vi "save.vi"(8 "error in (no error)":errorcluster caption="entrée d'erreur (pas d'erreur)", 11 "Model.lvclass":refnum<class "Model.lvclass">) -> (0 "error out":errorcluster caption="sortie d'erreur", 2 "filename":string, 3 "Model.lvclass 2":refnum<class "Model.lvclass">)   [LabVIEW 2020, in "Model.lvclass"]
doc: "Save a trained model"
uses:
  Model.lvclass
  C:/Users/cipop/TDF Dropbox/2_Technologies de France/1 - Services et Etudes/PLAIY/2 - DEV/PLAIYLAB/code/Python/Python.lvclass
  Model.lvclass/Model.ctl
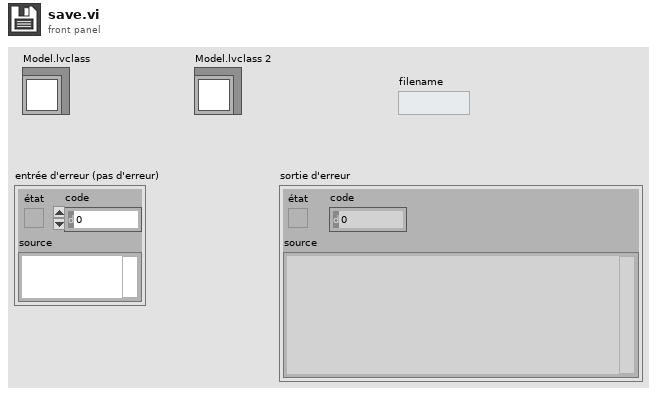
[diagram p1: front panel]
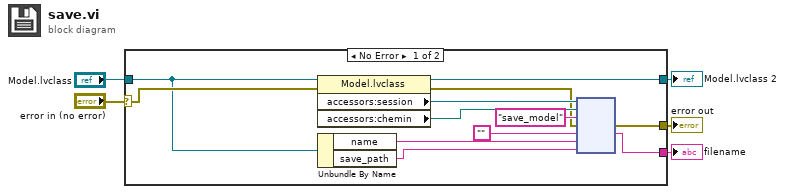
[diagram p0: block diagram]
diagram:
  n1 = case shown="No Error" "error in (no error)" {
    selector: "error in (no error)" -> [w15 w19]
    tunnel: [w16 w19] -> w4
    tunnel: [w12 w18] -> w2
    tunnel: "Model.lvclass" -> [w9 w18]
    tunnel: [w11 _] -> w1
    frame No Error {
      n2 = property class="Model.lvclass"(reference=w9, error in=w15) -> (reference out=w12:refnum<class "Model.lvclass">, error out=w10:errorcluster, "accessors:session"=w14:refnum<k35>, "accessors:chemin"=w13:path)
      n3 = Unbundle By Name(w9) -> ("name"=w7:string, "save_path"=w6:string)
      n4 = node(w14, w13, "save_model" ("nom de la fonction"), w10, "", w7, w6) -> (w16:errorcluster, w11:string)  [unwired: 2 in, 3 out]
    }
    frame Error {
    }
  }
  "error out" <- w4
  "Model.lvclass 2" <- w2
  "filename" <- w1
